vi "Sgl_NoneModifing.vi"(5 "Error In":errorcluster) -> (19 "Error Out":errorcluster)   [LabVIEW 2020, in "SingletonTemplate.lvclass"]
uses:
  SingletonTemplate.lvclass
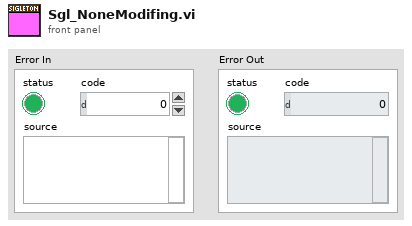
[diagram p1: front panel]
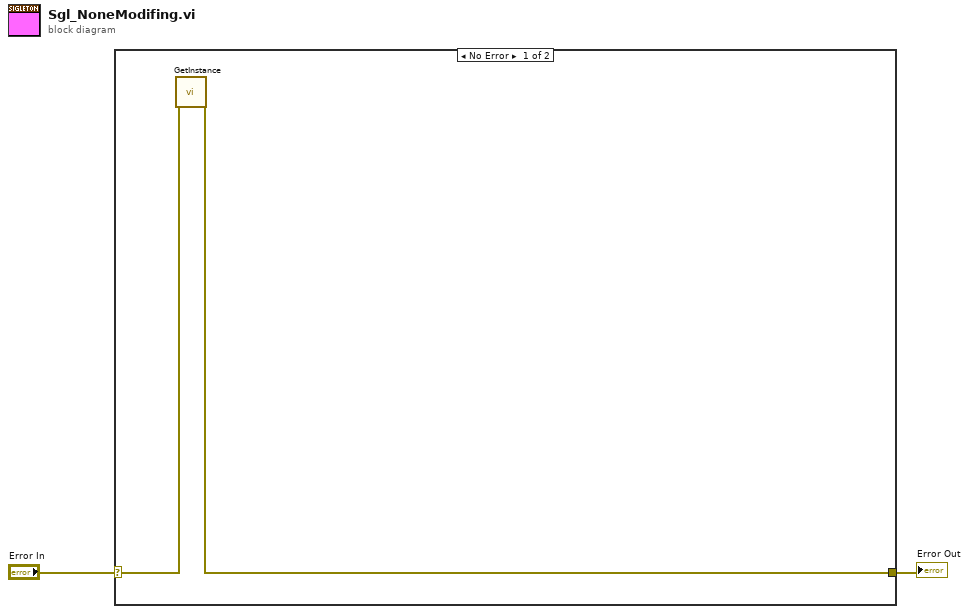
[diagram p0: block diagram]
diagram:
  n1 = case shown="No Error" "Error In" {
    selector: "Error In" -> [w4 w5]
    tunnel: [w3 w5] -> w1
    frame No Error {
      n2 = call "GetInstance.vi"("error in (no error)"=w4) -> ("error out"=w3:errorcluster)  [unwired: 17 in, 1 out]
    }
    frame Error {
    }
  }
  "Error Out" <- w1
